vi "PID Derivative Control start.vi"(0 "Temp In (deg C)":dbl format="%.2f", 7 "Control Parameters":T1={"Setpoint"=50.0, "Control Bandwidth"=4.0, "Integral Time"=30.0, "Int\nON"=TRUE, "Derivative Tme"=0.5, "Der\nON"=TRUE, "Settle Bandwidth"=1.0, "Settle Time"=30.0} {"Settle Time" step=1.0; "Settle Bandwidth" step=0.01; "Derivative Tme" step=0.01; "Integral Time" step=1.0; "Control Bandwidth" step=0.1; "Setpoint" step=0.1}, 9 "reset":bool, 11 "delta t":dbl format="%.2f") -> (8 "Derivative Power":dbl format="%.2f")   [LabVIEW 2019]
doc: "Subvi \nthis does the derivative portion of the main PID controller \n\nJuan Gamez \nP3600\nCSUSB"
uses:
  typedefs/PID control parameters.ctl
panel:
  # "PID\nDerivative\nPower\nControl"
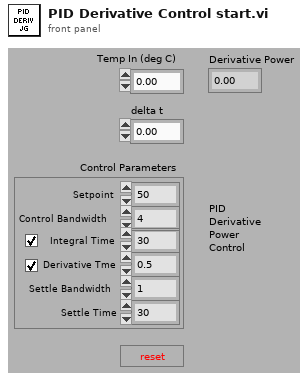
[diagram p1: front panel]
types:
  T1 = typedef "PID control parameters.ctl" = cluster{"Setpoint":dbl, "Control Bandwidth":dbl, "Integral Time":dbl, "Int\nON":bool, "Derivative Tme":dbl, "Der\nON":bool, "Settle Bandwidth":dbl, "Settle Time":dbl}
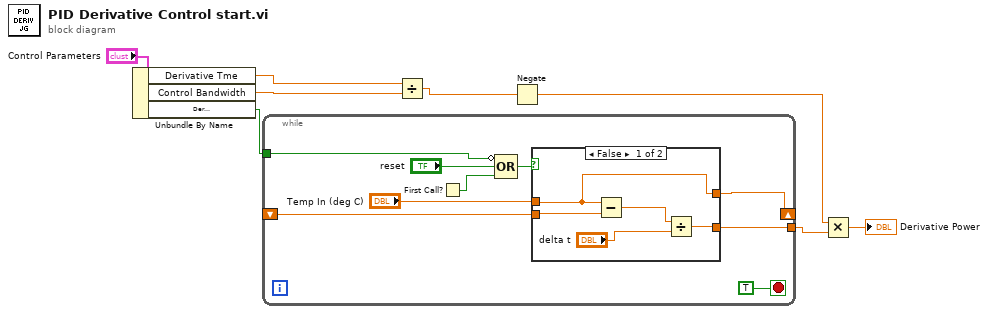
[diagram p0: block diagram]
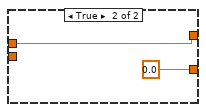
[diagram p2: hidden frame]
diagram:
  n1 = Unbundle By Name("Control Parameters") -> ("Derivative Tme"=w4:dbl, "Control Bandwidth"=w5:dbl, "Der\nON"=w7:bool)
  n2 = while {
    tunnel: w7 -> [w15]
    shift-right: [w12] -> _
    shift-left: _ -> [w10]
    tunnel: [w11] -> w6
    stop <- TRUE stop-if-true
    n3 = First Call?() -> (First Call?: T/F=w17:bool)
    n4 = Compound Arithmetic op=OR(invert w15, "reset", w17) -> (w14:bool)
    n5 = case shown="False" w14 {
      tunnel: [w18 w24] -> w12
      tunnel: "Temp In (deg C)" -> [w18 w24]
      tunnel: [w19 0.0 ("Derivative Power")] -> w11
      tunnel: w10 -> [w22 _]
      frame False {
        n6 = Subtract(x=w18, y=w22) -> (x-y=w20:dbl)
        n7 = Divide(x=w20, y="delta t") -> (x/y=w19:dbl)
      }
      frame True {
      }
    }
  }
  n8 = Divide(x=w4, y=w5) -> (x/y=w3:dbl)
  n9 = Negate(x=w3) -> (-x=w2:dbl)
  n10 = Multiply(x=w2, y=w6) -> (x*y=→"Derivative Power":dbl)
